vi "SystemTime_GetTimeZone.vi"(8 "Fehler (Eingang, kein Fehler)":errorcluster caption="Error_In", 11 "OXYGEN Ref In":refnum<visa-resource-name>) -> (0 "Fehler (Ausgang)":errorcluster caption="Error_Out", 1 "communication_data":T1, 2 "UTC offset in h":dbl, 3 "OXYGEN Ref Out":refnum<visa-resource-name>)   [LabVIEW 2020, in "OXYGEN_Datastream.lvlib"]
doc: "Queries the system time zone."
uses:
  OXYGEN_Datastream.lvlib
  TypeDefs/Cluster_RawCommData.ctl
  <vilib>/regexp/Match Regular Expression.xnode
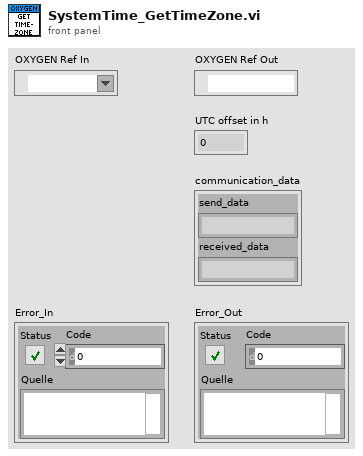
[diagram p1: front panel]
types:
  T1 = typedef "OXYGEN_Datastream.lvlib/Cluster_RawCommData.ctl" = cluster{"send_data":string, "received_data":string}
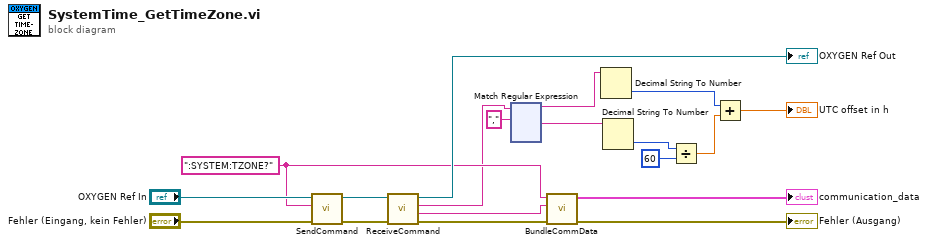
[diagram p0: block diagram]
diagram:
  w7 = ":SYSTEM:TZONE?" ("Schreibpuffer")
  n1 = call "SendCommand.vi"("error in (no error)"="Fehler (Eingang, kein Fehler)", "String to Send"=w7, "OXY_SCPI Reseource In"="OXYGEN Ref In") -> ("error out"=w9:errorcluster, "OXY_SCPI Reseource Out"=w8:refnum<visa-resource-name>)  [unwired: 7 in]
  n2 = call "ReceiveCommand.vi"("error in (no error)"=w9, "OXY_SCPI Reseource In"=w8) -> ("error out"=w5:errorcluster, "received Data with Header"=w1:string, "received Data"=w3:string, "OXY_SCPI Reseource Out"=→"OXYGEN Ref Out":refnum<visa-resource-name>)  [unwired: 6 in]
  n3 = xnode "Match Regular Expression"("input string"=w3, "regular expression"=",") -> ("before match"=w17:string, "after match"=w18:string)  [unwired: 4 in, 3 out]
  n4 = call "BundleCommData.vi"("error in (no error)"=w5, "received_data"=w1, "send_data"=w7) -> ("error out"=→"Fehler (Ausgang)":errorcluster, "communication_data"=→"communication_data":T1)  [unwired: 7 in]
  n5 = Decimal String To Number(string=w17) -> (number=w14:i32)  [unwired: 2 in, 1 out]
  n6 = Decimal String To Number(string=w18) -> (number=w16:i32)  [unwired: 2 in, 1 out]
  n7 = Divide(x=w16, y=60) -> (x/y=w13:dbl)
  n8 = Add(x=w14, y=w13) -> (x+y=→"UTC offset in h":dbl)
